vi "dfd_Get TF Render Coef.vi"(7 "type (FLP)":enum16{"FLP", "FXP"}(ring), 8 "error in (no error)":errorcluster, 9 "display format":u16(ring) items=["Expanded Form", " Second Order Sections"], 11 "filter in":T3={"mSRate_Fs"=1.0, "mSRate_Version"="1.0", "mSRate_Comments"="", "mSRate_OrgCoef"={"type"=enum."Undefined", "gain"=1.0, "coef a (k)"=[], "coef b (v)"=[]}, "mSRate_CurCoef"={"type"=enum."Undefined", "gain"=1.0, "coef a (k)"=[], "coef b (v)"=[]}, "mSRate_Quantized?"=FALSE, "mSRate_QCoef"={"type"=enum."Undefined", "gain"=1.0, "coef a (k)"=[], "coef b (v)"=[]}, "mSRate_QSettings"=[], "mSRate_Order"=0, "mSRate_Scaling"={"mSRate_ScaleByPowerOf2?"=FALSE, "mSRate_ScaleType"=enum."No Norm"}} {"mSRate_QSettings"."source" items=["Coef a/k"=0, "Coef b/v"=7, "Input"=1, "Output"=2, "Multiplicand"=3, "Product"=4, "Sum"=5, "Delay"=6, "Gain"=8]}) -> (0 "error out":errorcluster, 1 "display format":u16(ring) items=["Expanded Form", " Second Order Sections"], 3 "filter coef":T1={"type"=enum."Undefined", "gain"=1.0, "coef a (k)"=[], "coef b (v)"=[]})   [LabVIEW 2017, in "NI_DigFilter_Process.lvlib"]
uses:
  <vilib>/addons/Digital Filter Design/NI_DigFilter_Process.lvlib
  <vilib>/addons/Digital Filter Design/_Objects.llb/DFD Filter Obj.ctl
  <vilib>/addons/Digital Filter Design/_Objects.llb/DFD Filter Coef.ctl
  <vilib>/addons/Digital Filter Design/_Objects.llb/DFD Filter Structure Type Selector.ctl
  <vilib>/addons/Digital Filter Design/_Objects.llb/dfd_Internal Quantization Settings.ctl
  <vilib>/addons/Digital Filter Design/_Objects.llb/dfd_Internal Quantization Srcs.ctl
  <vilib>/addons/Digital Filter Design/_Objects.llb/DFD Coef Norm Type.ctl
  <vilib>/addons/Digital Filter Design/_Objects.llb/DFD Filter Structure Form Id.ctl
  <vilib>/addons/Digital Filter Design/NI_DigFilterLicensed.lvlib
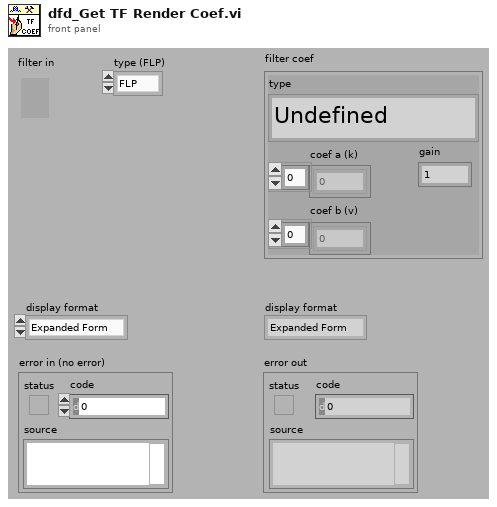
[diagram p1: front panel]
types:
  T1 = typedef "NI_DigFilterLicensed.lvlib/DFD Filter Coef.ctl" = cluster{"type":T2, "gain":dbl, "coef a (k)":dbl[], "coef b (v)":dbl[]}
  T2 = typedef "NI_DigFilterLicensed.lvlib/DFD Filter Structure Type Selector.ctl" = enum16{"Undefined", "FIR Direct Form", "FIR Direct Form Transposed", "FIR Symmetric", "FIR Antisymmetric", "IIR Direct Form I", "IIR Direct Form I Transposed", "IIR Direct Form II", "IIR Direct Form II Transposed", "IIR Cascaded Second Order Sections Form I", "IIR Cascaded Second Order Sections Form I Transposed", "IIR Cascaded Second Order Sections Form II", "IIR Cascaded Second Order Sections Form II Transposed", "Lattice Allpass (basic sections)", "Lattice Allpass (one multiplier sections)", "Lattice Allpass (normalized sections)", "Lattice AR (basic sections)", "Lattice AR (one multiplier sections)", "Lattice AR (normalized sections)", "Lattice MA (minimum phase)", "Lattice MA (maximum phase)", "Lattice ARMA (basic sections)", "Lattice ARMA (one multiplier sections)", "Lattice ARMA (normalized sections)"}
  T3 = typedef "NI_DigFilterLicensed.lvlib/DFD Filter Obj.ctl" = cluster{"mSRate_Fs":dbl, "mSRate_Version":string, "mSRate_Comments":string, "mSRate_OrgCoef":T1, "mSRate_CurCoef":T1, "mSRate_Quantized?":bool, "mSRate_QCoef":T1, "mSRate_QSettings":T4[], "mSRate_Order":i32, "mSRate_Scaling":cluster{"mSRate_ScaleByPowerOf2?":bool, "mSRate_ScaleType":T6}}
  T4 = typedef "NI_DigFilterLicensed.lvlib/dfd_Internal Quantization Settings.ctl" = cluster{"source":T5, "wl":i16, "iwl":i16, "overflow mode":enum16{"Saturation", "Wrap"}, "rounding mode":enum16{"Nearest", "Truncation"}, "signed?":bool}
  T5 = typedef "NI_DigFilterLicensed.lvlib/dfd_Internal Quantization Srcs.ctl" = u16
  T6 = typedef "NI_DigFilterLicensed.lvlib/DFD Coef Norm Type.ctl" = enum16{"No Norm", "Time Domain 1-Norm", "Time Domain 2-Norm", "Time Domain Inf-Norm"}
  T7 = typedef "NI_DigFilterLicensed.lvlib/DFD Filter Structure Form Id.ctl" = enum16{"Undefined", "Direct Form", "SOS Form", "Lattice Form"}
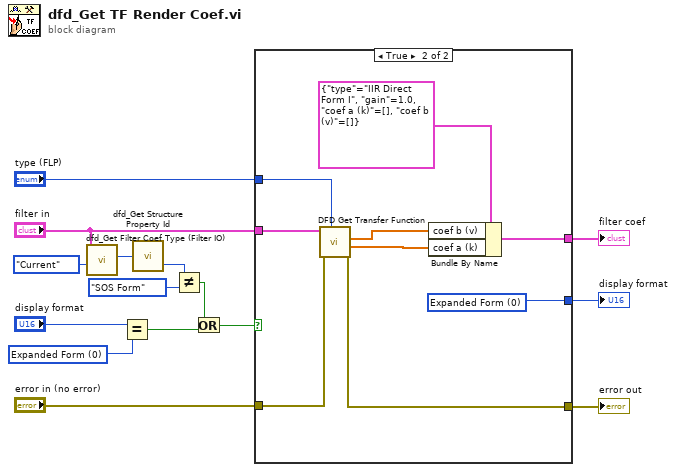
[diagram p0: block diagram]
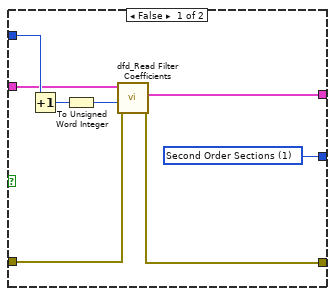
[diagram p2: hidden frame]
diagram:
  w3 = u16 0 items=["Expanded Form", " Second Order Sections"] ("display format")
  n1 = call <vilib>:"dfd_Get Filter Coef Type (Filter IO).vi"("coef source"=enum16{"Original", "Current", "Quantized"}."Current", "filter in"="filter in") -> ("type"=w9:T2)  [unwired: 1 in, 8 out]
  n2 = Equal?(x="display format", y=w3) -> (x = y?=w6:bool)
  n3 = call <vilib>:"dfd_Get Structure Property Id.vi"("structure type"=w9) -> ("filter structure form id"=w8:T7)  [unwired: 1 out]
  n4 = Not Equal?(x=w8, y=DFD_Filter_Structure_Form_Id."SOS Form") -> (x != y?=w5:bool)
  n5 = Or(x=w5, y=w6) -> (x .or. y?=w4:bool)
  n6 = case shown="True" w4 {
    tunnel: "filter in" -> [w22 w32]
    tunnel: "type (FLP)" -> [w23 w31]
    tunnel: [w21 w28] -> w14
    tunnel: [w18 w26] -> w13
    tunnel: "error in (no error)" -> [w17 w25]
    tunnel: [w16 w24] -> w1
    frame False {
      w18 = u16 1 items=["Expanded Form", " Second Order Sections"] ("display format")
      n7 = Increment(x=w23) -> (x+1=w20:enum16{"FLP", "FXP"})
      n8 = To Unsigned Word Integer(number=w20) -> (unsigned 16bit integer=w19:u16)
      n9 = call <vilib>:"dfd_Read Filter Coefficients.vi"("error in (no error)"=w17, "coef source"=w19, "filter in"=w22) -> ("error out"=w16:errorcluster, "filter coef"=w21:T1)  [unwired: 7 out]
    }
    frame True {
      w26 = u16 0 items=["Expanded Form", " Second Order Sections"] ("display format")
      n10 = call <vilib>:"DFD Get Transfer Function.vi"("type (FLP)"=w31, "error in (no error)"=w25, "filter in"=w32) -> ("error out"=w24:errorcluster, "denominator"=w29:dbl[], "numerator"=w30:dbl[])  [unwired: 6 out]
      n11 = Bundle By Name(cluster=T1 {"type"=enum."IIR Direct Form I", "gain"=1.0, "coef a (k)"=[], "coef b (v)"=[]} ("filter coef"), "coef b (v)"=w30, "coef a (k)"=w29) -> (w28:T1)
    }
  }
  "filter coef" <- w14
  "display format" <- w13
  "error out" <- w1
